vi "Actuator Point DAO.vi"(5 "section":string="Auto Balance Error", 7 "Config Ref  In":T3, 8 "error in (no error)":errorcluster, 9 "Point In":T2, 10 "LBCB Number":T1, 11 "Actions":T4) -> (0 "error out":errorcluster, 1 "Point Out":T2, 6 "Config Ref Out":T3)   [LabVIEW 2009]
uses:
  Metadata/Persistant DAO Actions.ctl
  Metadata/Actuator Point.ctl
  <vilib>/Utility/config.llb/Config Data RefNum.ctl
  Metadata/LBCB Number.ctl
  <vilib>/Utility/config.llb/NI_LVConfig.lvlib
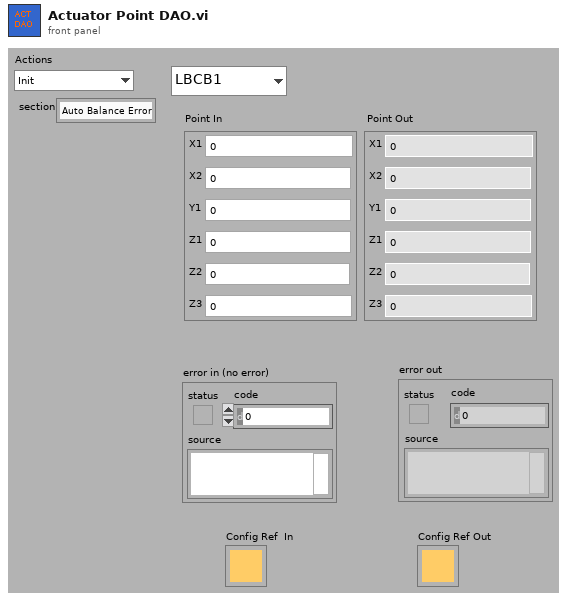
[diagram p1: front panel]
types:
  T1 = typedef "LBCB Number.ctl" = enum16{"LBCB1", "LBCB2"}
  T2 = typedef "Actuator Point.ctl" = cluster{"X1":dbl, "X2":dbl, "Y1":dbl, "Z1":dbl, "Z2":dbl, "Z3":dbl}
  T3 = typedef "NI_LVConfig.lvlib/Config Data RefNum.ctl" = refnum<k1>
  T4 = typedef "Persistant DAO Actions.ctl" = enum16{"Init", "Get", "Set", "Load", "Save"}
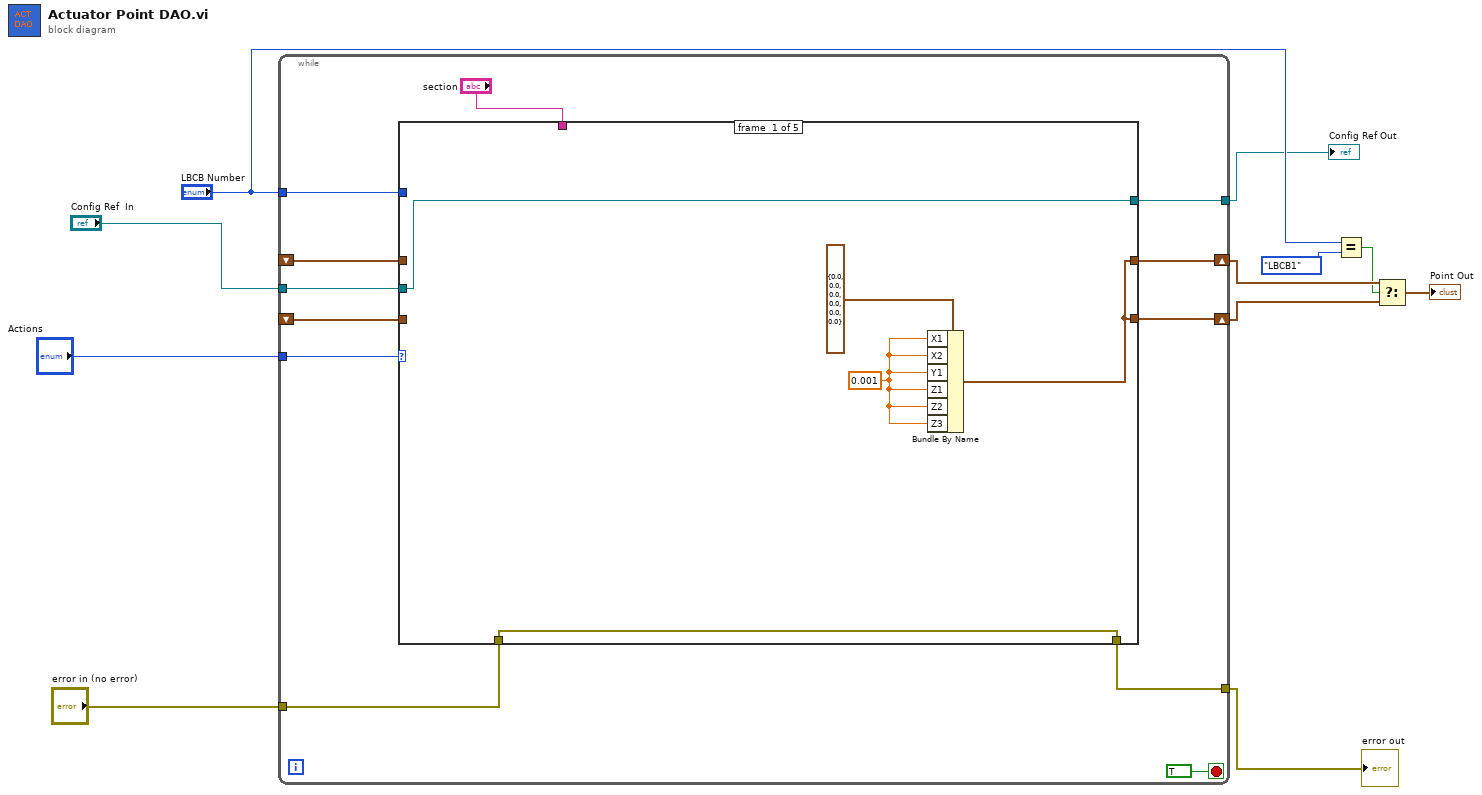
[diagram p0: block diagram]
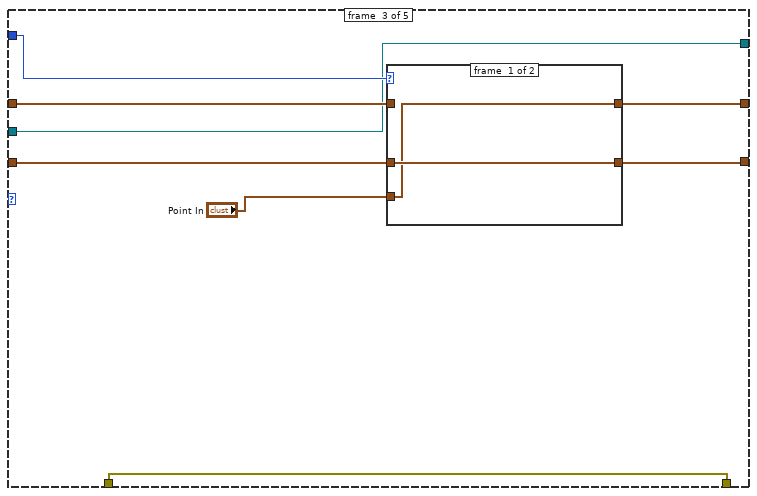
[diagram p3: hidden frame]
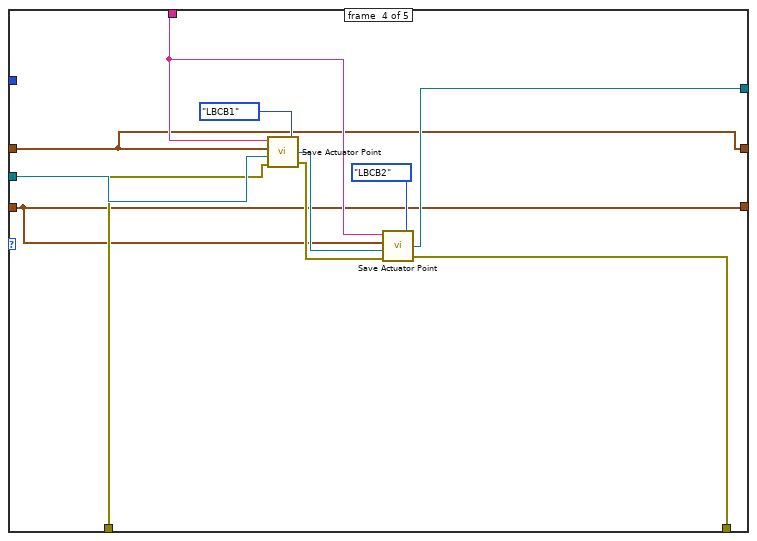
[diagram p5: hidden frame]
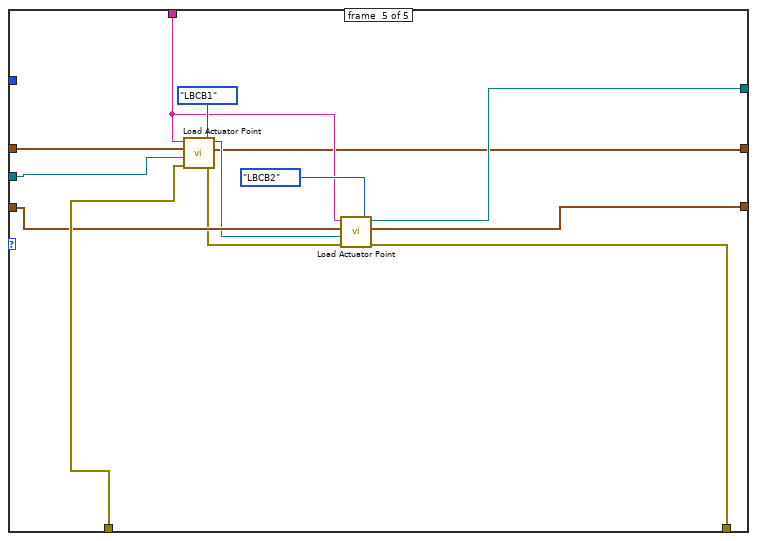
[diagram p6: hidden frame]
diagram:
  n1 = while {
    tunnel: "Actions" -> [w22]
    tunnel: "Config Ref  In" -> [w21]
    tunnel: "error in (no error)" -> [w19]
    tunnel: [w18] -> w1
    tunnel: [w17] -> w2
    shift-right: [w16] -> w8
    shift-left: _ -> [w15]
    tunnel: "LBCB Number" -> [w14]
    shift-right: [w13] -> w7
    shift-left: _ -> [w12]
    stop <- TRUE stop-if-true
    n2 = case shown="\"Init\"" w22 {
      tunnel: "section" -> [_ _ _ w51 w62]
      tunnel: w21 -> [w28 w30 w34 w55 w68]
      tunnel: w19 -> [w25 w29 w33 w54 w67]
      tunnel: [w28 w30 w34 w48 w59] -> w18
      tunnel: [w25 w29 w33 w47 w58] -> w17
      tunnel: [w26 w32 w35 w46 w57] -> w16
      tunnel: w15 -> [_ w32 w39 w46 w66]
      tunnel: w14 -> [_ _ w40 _ _]
      tunnel: [w26 w31 w36 w45 w56] -> w13
      tunnel: w12 -> [_ w31 w38 w45 w63]
      frame #0 {
        w24 = 0.001 ("X1")
        n3 = Bundle By Name(cluster=T2 {"X1"=0.0, "X2"=0.0, "Y1"=0.0, "Z1"=0.0, "Z2"=0.0, "Z3"=0.0} ("Auto Balance Increment"), "X1"=w24, "X2"=w24, "Y1"=w24, "Z1"=w24, "Z2"=w24, "Z3"=w24) -> (w26:T2)
      }
      frame #1 {
      }
      frame #2 {
        n4 = case shown="\"LBCB2\"" w40 {
          tunnel: w39 -> [_ w44]
          tunnel: w38 -> [w42 _]
          tunnel: "Point In" -> [w41 w43]
          tunnel: [w41 w44] -> w35
          tunnel: [w42 w43] -> w36
          frame #0 {
          }
          frame #1 {
          }
        }
      }
      frame #3 {
        n5 = call "Save Actuator Point.vi"("LBCB Number"=LBCB_Number."LBCB1", "error in (no error)"=w54, "refnum"=w55, "Input Cluster"=w46, "section"=w51) -> ("error out"=w50:errorcluster, "refnum out"=w49:T3)
        n6 = call "Save Actuator Point.vi"("LBCB Number"=LBCB_Number."LBCB2", "error in (no error)"=w50, "refnum"=w49, "Input Cluster"=w45, "section"=w51) -> ("error out"=w47:errorcluster, "refnum out"=w48:T3)
      }
      frame #4 {
        n7 = call "Load Actuator Point.vi"("LBCB Number"=LBCB_Number."LBCB1", "error in (no error)"=w67, "refnum"=w68, "Input Cluster"=w66, "section"=w62) -> ("error out"=w60:errorcluster, "Output Cluster"=w57:T2, "refnum out"=w61:T3)
        n8 = call "Load Actuator Point.vi"("LBCB Number"=LBCB_Number."LBCB2", "error in (no error)"=w60, "refnum"=w61, "Input Cluster"=w63, "section"=w62) -> ("error out"=w58:errorcluster, "Output Cluster"=w56:T2, "refnum out"=w59:T3)
      }
    }
  }
  "error out" <- w2
  "Config Ref Out" <- w1
  n9 = Equal?(x="LBCB Number", y=LBCB_Number."LBCB1") -> (x = y?=w6:bool)
  n10 = Select(t=w8, s=w6, f=w7) -> (s? t:f=→"Point Out":T2)
